vi "add lengtou2 set position(SubVI).vi"(6 "字符串":string) -> (0 "布尔 3":bool, 2 "连接的字符串":string)   [LabVIEW 2019, in "Add Seq.lvlib"]
uses:
  Add Seq.lvlib
panel:
  in  "cancel":bool
  in  "ok":bool
  in  "Speed":i32 min=0 max=14
  in  "Position":dbl=2.0 min=0.0 max=400.0
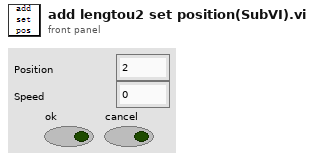
[diagram p1: front panel]
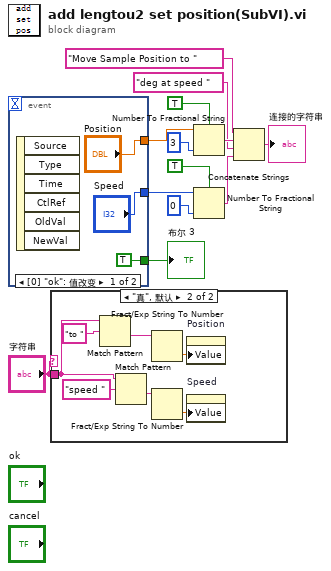
[diagram p0: block diagram]
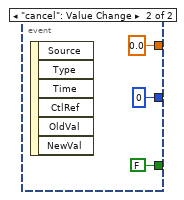
[diagram p3: hidden frame]
diagram:
  n1 = event shown="[0] \"ok\": 值改变" {
    selector: _ -> [_ _]
    dyn-events: _ -> [_ _]
    timeout: _ -> [_ _]
    tunnel: ["Speed" 0 ("Rate输入")] -> w4
    tunnel: ["Position" 0.0 ("Field")] -> w11
    tunnel: [TRUE FALSE] -> w13
    event "ok": Value Change {
      n2 = event-data() -> ()  [unwired: 1 in, 6 out]
    }
    event "cancel": Value Change {
      n3 = event-data() -> ()  [unwired: 1 in, 6 out]
    }
  }
  "布尔 3" <- w13
  n4 = case shown="\"真\", 默认" "字符串" {
    tunnel: "字符串" -> [_ w24]
    frame "" {
    }
    frame "真", Default {
      n5 = Match Pattern(string=w24, regular expression="to " ("正则表达式")) -> (after substring=w26:string)  [unwired: 1 in, 3 out]
      n6 = Match Pattern(string=w24, regular expression="speed " ("正则表达式")) -> (after substring=w22:string)  [unwired: 1 in, 3 out]
      n7 = Fract/Exp String To Number(string=w26) -> (number=w20:dbl)  [unwired: 3 in, 1 out]
      n8 = Fract/Exp String To Number(string=w22) -> (number=w21:dbl)  [unwired: 3 in, 1 out]
      n9 = property on="Position" class="DigNum (严格)"("Value"=w20) -> ()  [unwired: 2 in, 2 out]
      n10 = property on="Speed" class="DigNum (严格)"("Value"=w21) -> ()  [unwired: 2 in, 2 out]
    }
  }
  n11 = Number To Fractional String(use system decimal point (T)=TRUE ("使用系统小数点(T)"), number=w11, precision (6)=i16 3 ("精度(6)")) -> (F-format string=w9:string)  [unwired: 1 in]
  n12 = Number To Fractional String(use system decimal point (T)=TRUE ("使用系统小数点(T)"), number=w4, precision (6)=i16 0 ("精度(6)")) -> (F-format string=w3:string)  [unwired: 1 in]
  n13 = Concatenate Strings("Move Sample Position to " ("字符串"), w9, "deg at speed " ("字符串"), w3) -> (→"连接的字符串":string)
